vi "Example.vi"() -> ()   [LabVIEW 2015]
uses:
  Signals.ctl
  <vilib>/Erdos Miller/LV-Signals/create-xnode/LV-Create-Signals.xnode
  <vilib>/Erdos Miller/LV-Signals/read-write-xnode/LV-Read-Write-Signals.xnode
  <vilib>/Erdos Miller/LV-Signals/destroy-xnode/LV-Destroy-Signals.xnode
  test.lvlib
panel:
  out "String":string
  in  "Number":dbl=5.0 format="%#_13g"
  out "Values":T1
  in  "String":string
  in  "Array Index 2":i32=1
  in  "Array Index":i32
  in  "Stop Button":bool
  out "Array":cluster{"Array":cluster{"Number":dbl}[]}[](array[cluster])
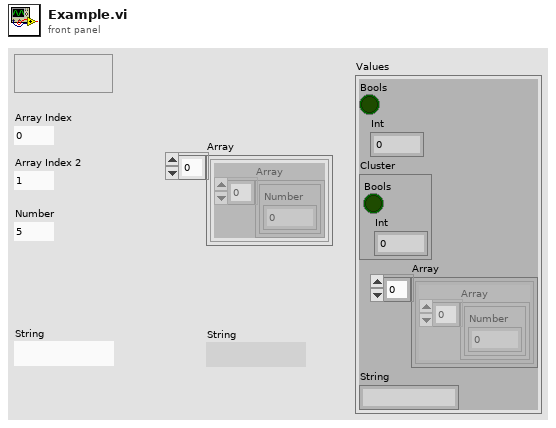
[diagram p1: front panel]
types:
  T1 = cluster{"Bools":bool, "Int":i32, "Cluster":cluster{"Bools":bool, "Int":i32}, "Array":cluster{"Array":cluster{"Number":dbl}[]}[], "String":string}
  T2 = cluster{"Bool":bool, "Int":i32, "Cluster":cluster{"Bool":bool, "Int":i32}, "Array":cluster{"Array":cluster{"Number":dbl}[]}[], "String":string}
  T3 = typedef "test.lvlib/Signals.ctl" = cluster{"DVR":refnum<data-value>, "Module Events":cluster{"Bool":refnum<user-event>, "Int":refnum<user-event>, "Cluster":refnum<user-event>, "Array":refnum<user-event>, "String":refnum<user-event>}}
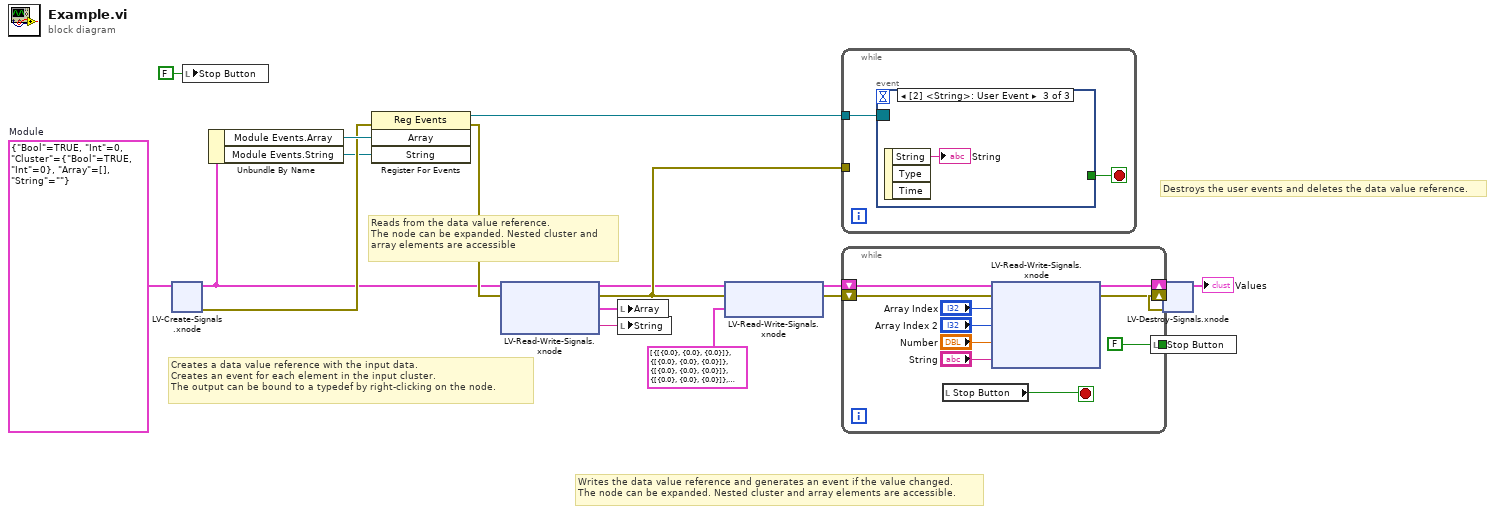
[diagram p0: block diagram]
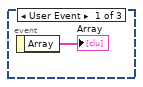
[diagram p2: hidden frame]
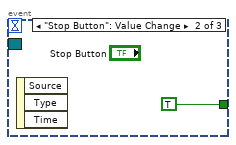
[diagram p3: hidden frame]
diagram:
  w2 = T2 {"Bool"=TRUE, "Int"=0, "Cluster"={"Bool"=TRUE, "Int"=0}, "Array"=[], "String"=""}  # Module
  # "Destroys the user events and deletes the data value reference."
  # "Writes the data value reference and generates an event if the value changed.\nThe node can be expanded. Nested cluster and array elements are accessible."
  # "Reads from the data value reference.\nThe node can be expanded. Nested cluster and\narray elements are accessible"
  # "Creates a data value reference with the input data.\nCreates an event for each element in the input cluster.\nThe output can be bound to a typedef by right-clicking on the node."
  n1 = xnode "LV-Create-Signals.xnode"("Values"=w2) -> ("Signals"=w1:T3, "Error Out"=w16:errorcluster)  [unwired: 1 in]
  n2 = local write "Stop Button"(FALSE ("Stop Button")) -> ()
  n3 = Unbundle By Name(w1) -> ("Module Events.Array"=w17:refnum<user-event>, "Module Events.String"=w7:refnum<user-event>)
  n4 = register-events(error in=w16, w17, w7) -> (reference out=w14:refnum<event-registration>, error out=w15:errorcluster)  [unwired: 1 in]
  n5 = xnode "LV-Read-Write-Signals.xnode"("Signals In"=w1, "Error In"=w15) -> ("Signals Out"=w9:T3, "Error Out"=w12:errorcluster, "Array"=w5:cluster{"Array":cluster{"Number":dbl}[]}[], "String"=w4:string)
  n6 = local write "Array"(w5) -> ()
  n7 = local write "String"(w4) -> ()
  n8 = xnode "LV-Read-Write-Signals.xnode"("Signals In"=w9, "Error In"=w12, "Array"=cluster{"Array":cluster{"Number":dbl}[]}[] [{"Array"=[{"Number"=0.0}, {"Number"=0.0}, {"Number"=0.0}]}, {"Array"=[{"Number"=0.0}, {"Number"=0.0}, {"Number"=0.0}]}, {"Array"=[{"Number"=0.0}, {"Number"=0.0}, {"Number"=0.0}]}, {"Array"=[{"Number"=0.0}, {"Number"=0.0}, {"Number"=0.0}]}, {"Array"=[{"Number"=0.0}, {"Number"=0.0}, {"Number"=0.0}]}]) -> ("Signals Out"=w13:T3, "Error Out"=w11:errorcluster)
  n9 = while {
    tunnel: w14 -> [w21]
    tunnel: w12 -> [_]
    stop <- w20 stop-if-true
    n10 = event shown="[2] <String>: User Event" {
      selector: w21 -> [_ _ _]
      dyn-events: _ -> [_ _ _]
      timeout: _ -> [_ _ _]
      tunnel: [_ TRUE _] -> w20
      event User Event {
        n11 = event-data() -> ("Array"=→"Array":cluster{"Array":cluster{"Number":dbl}[]}[])  [unwired: 1 in]
      }
      event "Stop Button": Value Change {
        n12 = event-data() -> ()  [unwired: 1 in, 3 out]
      }
      event User Event {
        n13 = event-data() -> ("String"=→"String":string)  [unwired: 1 in, 2 out]
      }
    }
  }
  n14 = while {
    shift-right: [w34] -> w19
    shift-left: w13 -> [w32]
    shift-right: [w33] -> w18
    shift-left: w11 -> [w31]
    tunnel: [FALSE] -> w8
    stop <- w30 stop-if-true
    n15 = local read "Stop Button"() -> (w30:bool)
    n16 = xnode "LV-Read-Write-Signals.xnode"("Signals In"=w32, "Error In"=w31, "Array[]"="Array Index", "Element.Array[]"="Array Index 2", "Element.Number"="Number", "String"="String") -> ("Signals Out"=w34:T3, "Error Out"=w33:errorcluster)
  }
  n17 = local write "Stop Button"(w8) -> ()
  n18 = xnode "LV-Destroy-Signals.xnode"("Signals"=w19, "Error In"=w18) -> ("Values"=→"Values":T2)  [unwired: 1 out]
